vi "Field_Step_AMI.vi"   [LabVIEW 2019]
uses:
  Monitors/Utility/Monitor Communication/AMI/AMI_Control.ctl
  Global/Global Variables/global.vi
  Global/Global Variables/Data_Display_global.vi
  Instrument_Setup.vi
types:
  T1 = typedef "AMI_Control.ctl" = cluster{"B AMI rate (T)":dbl, "AMI Set field":bool, "B AMI Setpoint (T)":dbl, "Phi AMI Setpoint (Deg) ":dbl, "Switch Heater":bool, "Y-Axis Setpoint (T)":dbl, "Y-Axis Rate (T/min)":dbl, "Z-Axis Setpoint (T)":dbl, "Z-Axis Rate (T/min)":dbl}
  T2 = typedef "AMI_cluster.ctl" = cluster{"Y Axis Status":enum16{"", "RAMPING", "HOLDING", "PAUSED", "MANUAL UP", "MANUAL DOWN", "ZEROING CURRENT", "QUENCH DETECTED", "HEATING SWITCH", "AT ZER0", "COOLING SWITCH"}, "Z Axis Status":enum16{"", "RAMPING", "HOLDING", "PAUSED", "MANUAL UP", "MANUAL DOWN", "ZEROING CURRENT", "QUENCH DETECTED", "HEATING SWITCH", "AT ZER0", "COOLING SWITCH"}, "Y-Axis (T)":dbl, "Y-Axis Setpoint (T)":dbl, "Y-Axis Rate (T/min)":dbl, "Z-Axis (T)":dbl, "Z-Axis Setpoint (T)":dbl, "Z-Axis Rate (T/min)":dbl, "B AMI rate (T)":dbl, "AMI Monitor":bool, "AMI Set field rates":bool, "AMI Set field":bool, "Switch Heater Y":bool, "Switch Heater Z":bool, "Switch Heater":bool, "B AMI (T)":dbl, "B AMI Setpoint (T)":dbl, "Phi AMI (Deg) ":dbl, "Phi AMI Setpoint (Deg) ":dbl}
  T3 = enum16{"", "RAMPING", "HOLDING", "PAUSED", "MANUAL UP", "MANUAL DOWN", "ZEROING CURRENT", "QUENCH DETECTED", "HEATING SWITCH", "AT ZER0", "COOLING SWITCH"}
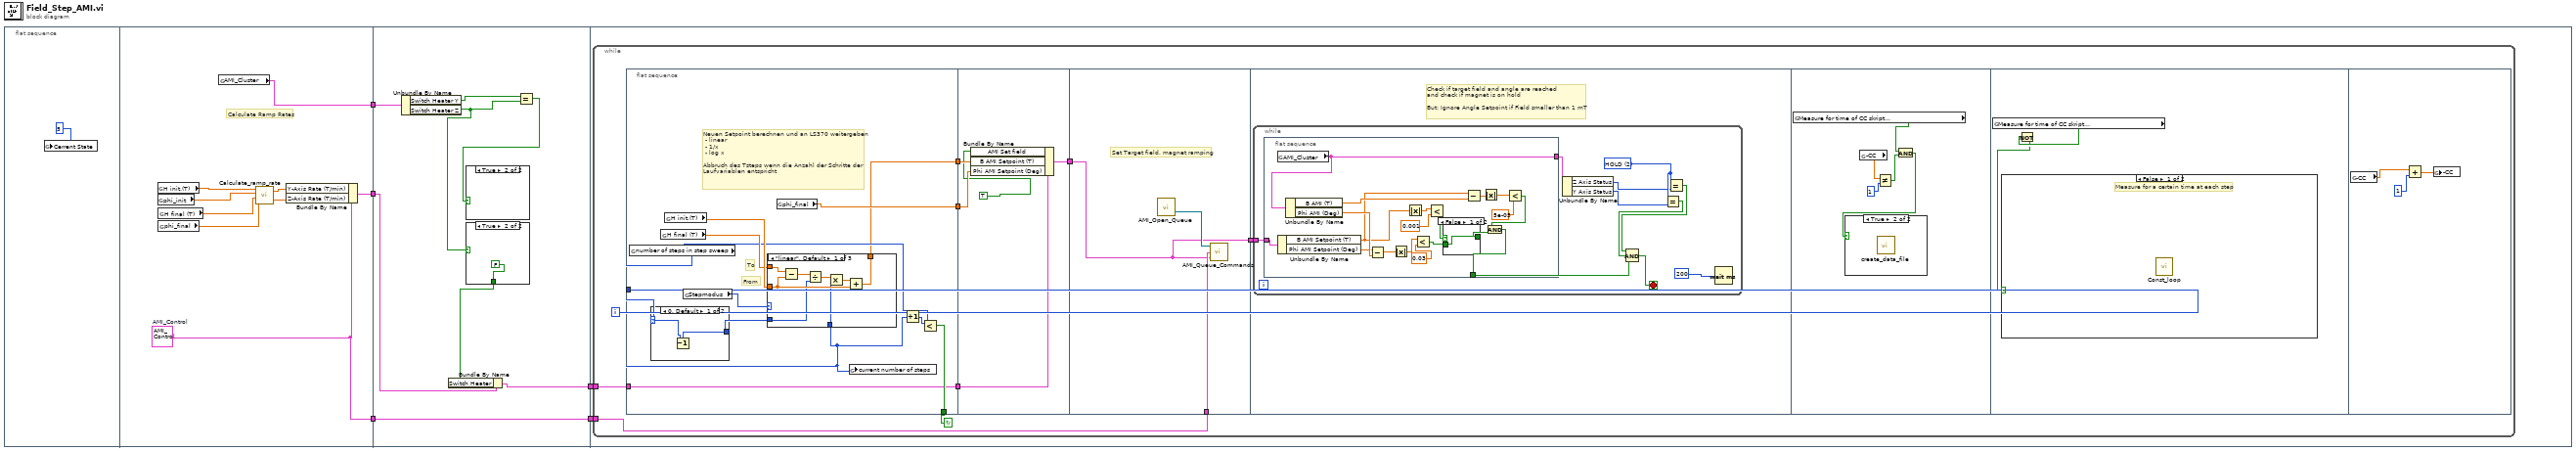
[diagram p0: block diagram]
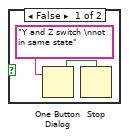
[diagram p2: hidden frame]
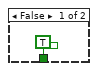
[diagram p3: hidden frame]
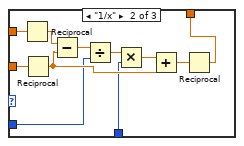
[diagram p5: hidden frame]
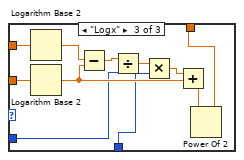
[diagram p6: hidden frame]
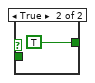
[diagram p7: hidden frame]
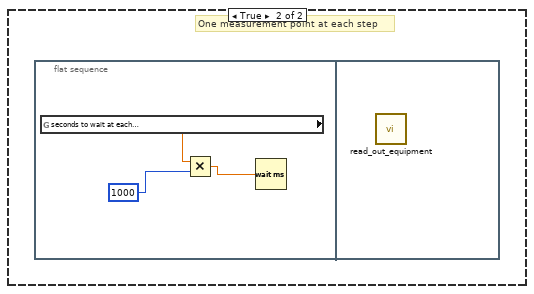
[diagram p9: hidden frame]
diagram:
  n1 = flat-sequence {
    tunnel: [w9] -> w5
    tunnel: [w8] -> w4
    tunnel: [w7] -> w1
    tunnel: w5 -> [w22]
    tunnel: w4 -> [w21]
    tunnel: [w17] -> w3
    tunnel: [w16] -> w2
    tunnel: w1 -> [w16]
    tunnel: w3 -> [w29]
    tunnel: w2 -> [w28]
    frame #0 {
      n2 = global write "global.vi" "Cerrent State"(5) -> ()
    }
    frame #1 {
      w7 = T1 {"B AMI rate (T)"=0.0, "AMI Set field"=FALSE, "B AMI Setpoint (T)"=0.0, "Phi AMI Setpoint (Deg) "=0.0, "Switch Heater"=FALSE, "Y-Axis Setpoint (T)"=0.0, "Y-Axis Rate (T/min)"=0.0, "Z-Axis Setpoint (T)"=0.0, "Z-Axis Rate (T/min)"=0.0}  # AMI_Control
      # "Calculate Ramp Rates"
      n3 = global read "global.vi" "H init.(T)"() -> (w15:dbl)
      n4 = global read "global.vi" "phi_init"() -> (w14:dbl)
      n5 = global read "global.vi" "H final (T)"() -> (w13:dbl)
      n6 = global read "global.vi" "phi_final"() -> (w12:dbl)
      n7 = global read "Data_Display_global.vi" "AMI_Cluster"() -> (w8:T2)
      n8 = call "Calculate_ramp_rate.vi"("Phi (Deg)"=w12, "H_final (T)"=w13, "Phi_init (Deg)"=w14, "H_init (T)"=w15) -> ("Z-Ramp"=w10:dbl, "Y-Ramp"=w11:dbl)  [unwired: 2 in]
      n9 = Bundle By Name(cluster=w7, "Y-Axis Rate (T/min)"=w11, "Z-Axis Rate (T/min)"=w10) -> (w9:T1)
    }
    frame #2 {
      n10 = Unbundle By Name(w21) -> ("Switch Heater Y"=w20:bool, "Switch Heater Z"=w18:bool)
      n11 = case shown="True" w18 {
        tunnel: [TRUE FALSE] -> w23
        frame False {
        }
        frame True {
        }
      }
      n12 = Bundle By Name(cluster=w22, "Switch Heater"=w23) -> (w17:T1)
      n13 = Equal?(x=w20, y=w18) -> (x = y?=w19:bool)
      n14 = case shown="True" w19 {
        frame False {
          n15 = One Button Dialog(message="Y and Z switch \nnot in same state") -> (true=w24:bool)  [unwired: 1 in]
          n16 = Stop(stop? (T)=w24) -> ()
        }
        frame True {
        }
      }
    }
    frame #3 {
      n17 = while {
        tunnel: w29 -> [w32]
        tunnel: w28 -> [w31]
        i -> [w38]
        stop <- w37 continue-if-true
        n18 = flat-sequence {
          tunnel: w38 -> [w43]
          tunnel: [w42] -> w37
          tunnel: [w41] -> w36
          tunnel: [w40] -> w35
          tunnel: [w39] -> w33
          tunnel: w32 -> [w39]
          tunnel: w36 -> [w87]
          tunnel: w35 -> [w86]
          tunnel: [w84] -> w34
          tunnel: w33 -> [w83]
          tunnel: w34 -> [w88]
          tunnel: w31 -> [w89]
          tunnel: [w88] -> w30
          tunnel: w30 -> [w91]
          frame #0 {
            # "Neuen Setpoint berechnen und an LS370 weitergeben\n - linear\n - 1/x\n - log x\n\nAbbruch des Tsteps wenn die Anzahl der Schritte der \nLaufvariablen entspricht"
            # "From"
            # "To"
            n19 = global read "global.vi" "number of steps in step sweep"() -> (w46:i32)
            n20 = case shown="0, Default" w46 {
              selector: w46 -> [w51 w52]
              tunnel: [w50 w52] -> w45
              frame 0, Default {
                n21 = Decrement(x=w51) -> (x-1=w50:i32)
              }
              frame 1 {
              }
            }
            n22 = global read "global.vi" "H final (T)"() -> (w48:dbl)
            n23 = global read "global.vi" "H init.(T)"() -> (w49:dbl)
            n24 = global read "Instrument_Setup.vi" "Stepmodus"() -> (w47:enum16{"linear", "1/x", "Logx"})
            n25 = case shown="\"linear\", Default" w47 {
              tunnel: w48 -> [w60 w70 w82]
              tunnel: w49 -> [w57 w71 w81]
              tunnel: [w55 w65 w74] -> w40
              tunnel: w45 -> [w54 w62 w73]
              tunnel: w43 -> [w53 w61 w72]
              frame "linear", Default {
                n26 = Subtract(x=w60, y=w57) -> (x-y=w59:dbl)
                n27 = Divide(x=w59, y=w54) -> (x/y=w58:dbl)
                n28 = Multiply(x=w58, y=w53) -> (x*y=w56:dbl)
                n29 = Add(x=w56, y=w57) -> (x+y=w55:dbl)
              }
              frame "1/x" {
                n30 = Reciprocal(x=w70) -> (1/x=w64:dbl)
                n31 = Reciprocal(x=w71) -> (1/x=w63:dbl)
                n32 = Subtract(x=w64, y=w63) -> (x-y=w69:dbl)
                n33 = Divide(x=w69, y=w62) -> (x/y=w68:dbl)
                n34 = Multiply(x=w68, y=w61) -> (x*y=w67:dbl)
                n35 = Add(x=w67, y=w63) -> (x+y=w66:dbl)
                n36 = Reciprocal(x=w66) -> (1/x=w65:dbl)
              }
              frame "Logx" {
                n37 = Logarithm Base 2(1:w82) -> (0:w80:dbl)
                n38 = Logarithm Base 2(1:w81) -> (0:w76:dbl)
                n39 = Subtract(x=w80, y=w76) -> (x-y=w79:dbl)
                n40 = Divide(x=w79, y=w73) -> (x/y=w78:dbl)
                n41 = Multiply(x=w78, y=w72) -> (x*y=w77:dbl)
                n42 = Add(x=w77, y=w76) -> (x+y=w75:dbl)
                n43 = Power Of 2(x=w75) -> (2^x=w74:dbl)
              }
            }
            n44 = global read "global.vi" "phi_final"() -> (w41:dbl)
            n45 = global write "Data_Display_global.vi" "current number of steps"(w43) -> ()
            n46 = Increment(x=w43) -> (x+1=w44:i32)
            n47 = Less?(x=w44, y=w46) -> (x < y?=w42:bool)
          }
          frame #1 {
            n48 = Bundle By Name(cluster=w83, "AMI Set field"=TRUE, "B AMI Setpoint (T)"=w86, "Phi AMI Setpoint (Deg)"=w87) -> (w84:T1)
          }
          frame #2 {
            # "Set Target field, magnet ramping"
            n49 = call "AMI_Open_Queue.vi"() -> ("queue out"=w90:refnum<queue>)  [unwired: 10 in, 1 out]
            n50 = call "AMI_Queue_Commands.vi"("AMI_Control"=w88, "Last Status"=w89, "Queue in"=w90) -> ()  [unwired: 1 out]
          }
          frame #3 {
            # "Check if target field and angle are reached\nand check if magnet is on hold\n\nBut: Ignore Angle Setpoint if Field smaller than 1 mT"
            n51 = while {
              tunnel: w91 -> [w92]
              stop <- w99 stop-if-true
              w98 = u16 2 items=["RAMP"=1, "HOLD"=2, "Paused"=3, "Manual Up"=4, "Manual Down"=5, "Zeroing Current"=6, "Quench Detected"=7, "At Zero"=8, "Heating Switch"=9, "Cooling Switch "=10] ("Ramping Mode")
              n52 = flat-sequence {
                tunnel: [w113] -> w100
                tunnel: [w105] -> w95
                tunnel: w92 -> [w104]
                frame #0 {
                  n53 = global read "Data_Display_global.vi" "AMI_Cluster"() -> (w105:T2)
                  n54 = Unbundle By Name(w104) -> ("B AMI Setpoint (T)"=w102:dbl, "Phi AMI Setpoint (Deg)"=w103:dbl)
                  n55 = Unbundle By Name(w105) -> ("B AMI (T)"=w107:dbl, "Phi AMI (Deg)"=w106:dbl)
                  n56 = Subtract(x=w103, y=w106) -> (x-y=w115:dbl)
                  n57 = Absolute Value(x=w115) -> (abs(x)=w116:dbl)
                  n58 = Absolute Value(x=w102) -> (abs(x)=w112:dbl)
                  n59 = Less?(x=w116, y=0.03) -> (x < y?=w108:bool)
                  n60 = Less?(x=w112, y=0.001) -> (x < y?=w110:bool)
                  n61 = case shown="False" w110 {
                    tunnel: [w121 TRUE] -> w109
                    tunnel: w108 -> [w121 _]
                    frame False {
                    }
                    frame True {
                    }
                  }
                  n62 = Subtract(x=w102, y=w107) -> (x-y=w119:dbl)
                  n63 = Absolute Value(x=w119) -> (abs(x)=w118:dbl)
                  n64 = Less?(x=w118, y=5e-05) -> (x < y?=w114:bool)
                  n65 = And(x=w114, y=w109) -> (x .and. y?=w113:bool)
                }
              }
              n66 = Unbundle By Name(w95) -> ("Z Axis Status"=w94:T3, "Y Axis Status"=w93:T3)
              n67 = Equal?(x=w98, y=w93) -> (x = y?=w97:bool)
              n68 = Equal?(x=w98, y=w94) -> (x = y?=w96:bool)
              n69 = Compound Arithmetic op=AND(w96, w97, w100) -> (w99:bool)
              n70 = Wait (ms)(milliseconds to wait=200) -> ()  [unwired: 1 out]
            }
          }
          frame #4 {
            n71 = global read "Instrument_Setup.vi" "Measure for time of CC skript\nat each field step point"() -> (w125:bool)
            n72 = global read "global.vi" "-CC"() -> (w127:dbl)
            n73 = Not Equal?(x=w127, y=1) -> (x != y?=w124:bool)
            n74 = And(x=w125, y=w124) -> (x .and. y?=w123:bool)
            n75 = case shown="True" w123 {
              frame False {
              }
              frame True {
                n76 = call "create_data_file.vi"() -> ()  [unwired: 3 in]
              }
            }
          }
          frame #5 {
            n77 = global read "Instrument_Setup.vi" "Measure for time of CC skript\nat each field step point"() -> (w129:bool)
            n78 = Not(x=w129) -> (.not. x?=w128:bool)
            n79 = case shown="False" w128 {
              frame False {
                # "Measure for a certain time at each step"
                n80 = call "Const_loop.vi"() -> ()  [unwired: 4 in]
              }
              frame True {
                # "One measurement point at each step"
                n81 = flat-sequence {
                  frame #0 {
                    n82 = global read "Instrument_Setup.vi" "seconds to wait at each\nfield step in a step sweep"() -> (w132:dbl)
                    n83 = Multiply(x=w132, y=u32 1000 ("milliseconds to wait")) -> (x*y=w130:dbl)
                    n84 = Wait (ms)(milliseconds to wait=w130) -> ()  [unwired: 1 out]
                  }
                  frame #1 {
                    n85 = call "read_out_equipment.vi"() -> ()  [unwired: 1 in]
                  }
                }
              }
            }
          }
          frame #6 {
            n86 = global read "global.vi" "-CC"() -> (w135:dbl)
            n87 = Add(x=w135, y=1) -> (x+y=w133:dbl)
            n88 = global write "global.vi" "-CC"(w133) -> ()
          }
        }
      }
    }
  }
